vi "Write.vi"   [LabVIEW 2018]
uses:
  <vilib>/eio/EIONode/EIONode.xnode
  <vilib>/rvi/eio/common/nirviEmuTemplateMethod_errors.vi
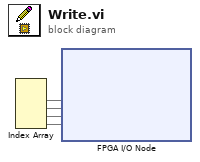
[diagram p0: block diagram]
diagram:
  n1 = Index Array() -> (array=w5:sgl[], element #1=w1, element #2=w2, element #3=w3, element #4=w4)  [unwired: 4 in]
  n2 = xnode "FPGA I/O Node"("00-04-9265/AO0"=w1, "00-04-9265/AO1"=w2, "00-04-9265/AO2"=w3, "00-04-9265/AO3"=w4) -> ()  [unwired: 5 in, 5 out]
